vi "FGV Read Central Message Logger.vi"(8 "Error In":errorcluster, 11 "CS++MessageLogger in":refnum<class "CS++MessageLogger.lvclass">) -> (0 "Error Out":errorcluster, 3 "CS++MessageLogger out":refnum<class "CS++MessageLogger.lvclass">)   [LabVIEW 2015, in "CS++Base.lvlib"]
doc: "Read FGV storing the central CS++MessageLogger object."
uses:
  CS++Base.lvlib
  Classes/CS++BaseClasses/MessageLogger/CS++MessageLogger.lvclass
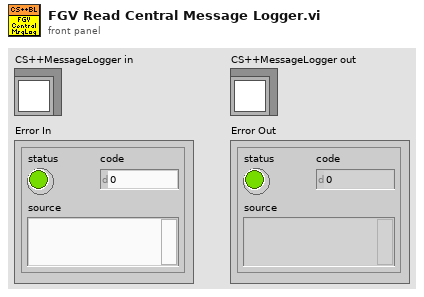
[diagram p1: front panel]
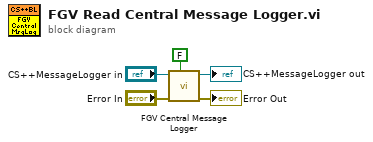
[diagram p0: block diagram]
diagram:
  n1 = call "FGV Central Message Logger.vi"("Write? (F)"=FALSE, "Error In"="Error In", "CS++MessageLogger in"="CS++MessageLogger in") -> ("Error Out"=→"Error Out":errorcluster, "CS++MessageLogger out"=→"CS++MessageLogger out":refnum<class "CS++MessageLogger.lvclass">)  [unwired: 7 in]
